vi "Find Salt.vi"(8 "error in (no error)":errorcluster, 11 "Content in":T1) -> (0 "error out":errorcluster, 1 "Salt":string, 2 "BDPW":T3, 3 "Content out":T1)   [LabVIEW 2021, in "VI-Hacker.lvlib"]
uses:
  VI-Hacker.lvlib
  TypeDefs/Content.ctl
  TypeDefs/Block.ctl
  TypeDefs/Block BDPW.ctl
  <vilib>/Utility/error.llb/Error Cluster From Error Code.vi
  <vilib>/ErrorRing/Error Ring.xnode
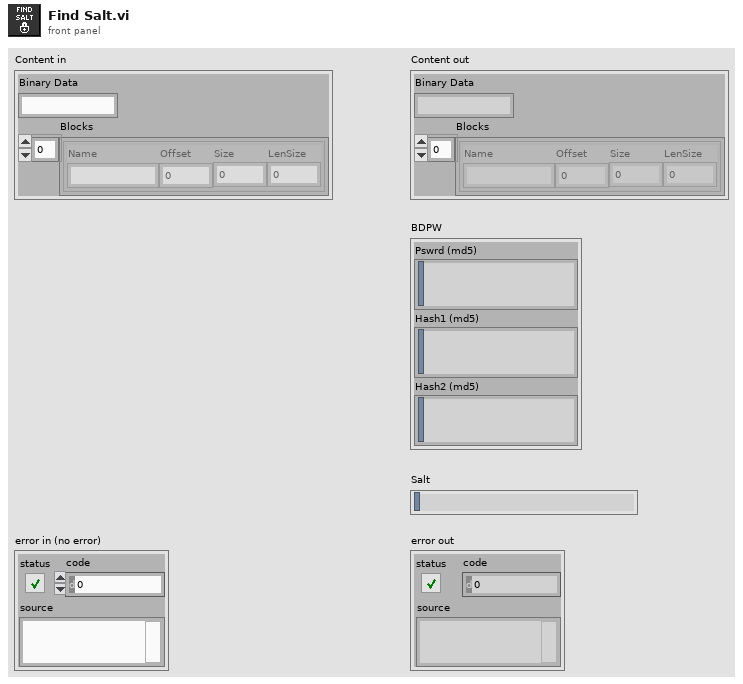
[diagram p1: front panel]
types:
  T1 = typedef "VI-Hacker.lvlib/Content.ctl" = cluster{"Binary Data":string, "Blocks":T2[]}
  T2 = typedef "VI-Hacker.lvlib/Block.ctl" = cluster{"Name":string, "Offset":i32, "Size":i32, "LenSize":i32}
  T3 = typedef "VI-Hacker.lvlib/Block BDPW.ctl" = cluster{"Pswrd (md5)":string, "Hash1 (md5)":string, "Hash2 (md5)":string}
  T4 = typedef "VI-Hacker.lvlib/Block vers.ctl" = cluster{"Version":cluster{"Major":u8, "Minor":u8, "Fix":u8, "Build":u8}, "Stage":enum8{"Development", "Alpha", "Beta", "Release"}, "Flags":u16, "VersionString":string, "VersionInfo":string}
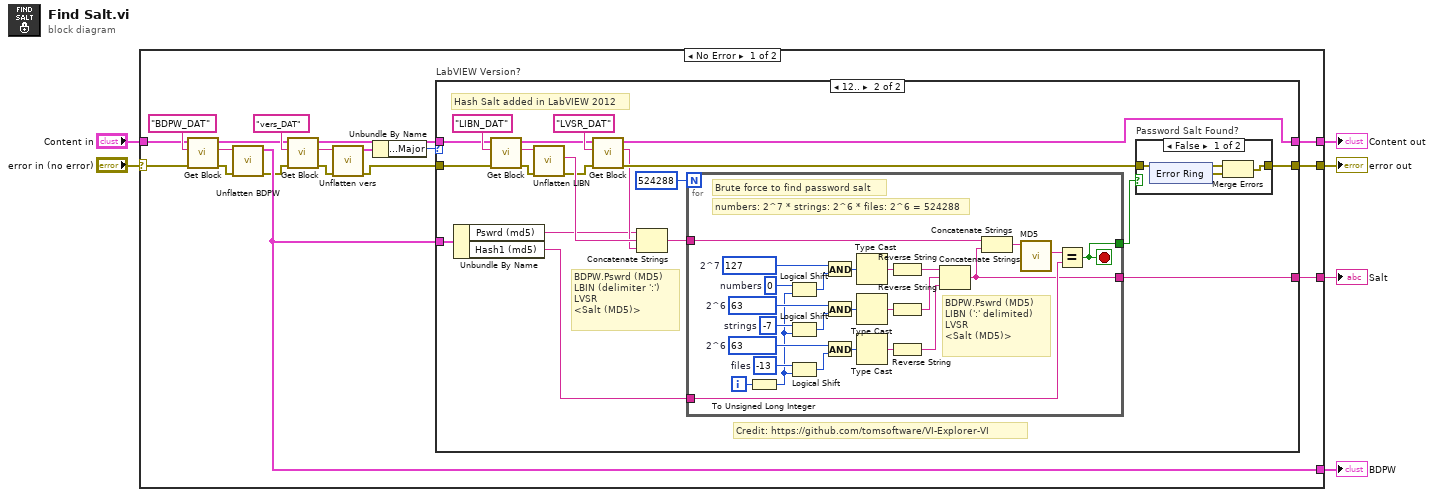
[diagram p0: block diagram]
diagram:
  n1 = case shown="No Error" "error in (no error)" {
    selector: "error in (no error)" -> [w13 w83]
    tunnel: [w24 w83] -> w6
    tunnel: [w23 _] -> w5
    tunnel: [w15 w82] -> w4
    tunnel: [w14 _] -> w3
    tunnel: "Content in" -> [w12 w82]
    frame No Error {
      n2 = call "Get Block.vi"("error in (no error)"=w13, "Block Name"="BDPW_DAT", "Content in"=w12) -> ("error out"=w19:errorcluster, "Data out"=w20:string, "Content out"=w11:T1)  [unwired: 4 in, 2 out]
      n3 = call "Unflatten BDPW.vi"("error in (no error)"=w19, "Data in"=w20) -> ("error out"=w10:errorcluster, "BDPW"=w14:T3)  [unwired: 8 in]
      n4 = call "Get Block.vi"("error in (no error)"=w10, "Block Name"="vers_DAT", "Content in"=w11) -> ("error out"=w18:errorcluster, "Data out"=w17:string, "Content out"=w8:T1)  [unwired: 4 in, 2 out]
      n5 = call "Unflatten vers.vi"("error in (no error)"=w18, "Data in"=w17) -> ("error out"=w9:errorcluster, "vers"=w16:T4)  [unwired: 8 in]
      n6 = Unbundle By Name(w16) -> ("Version.Major"=w7:u8)
      n7 = case "LabVIEW Version?" shown="12.." w7 {
        tunnel: [w26 w46] -> w24
        tunnel: [_ w45] -> w23
        tunnel: [w25 w33] -> w15
        tunnel: w14 -> [_ w32]
        tunnel: w9 -> [w26 w28]
        tunnel: w8 -> [w25 w27]
        frame ..11 {
          # "No salt in LabVIEW 2011 or before"
        }
        frame 12.. {
          # "Credit: https://github.com/tomsoftware/VI-Explorer-VI"
          # "BDPW.Pswrd (MD5)\nLBIN (delimiter ':')\nLVSR\n<Salt (MD5)>"
          # "Hash Salt added in LabVIEW 2012"
          n8 = Unbundle By Name(w32) -> ("Pswrd (md5)"=w35:string, "Hash1 (md5)"=w34:string)
          n9 = call "Get Block.vi"("error in (no error)"=w28, "Block Name"="LIBN_DAT", "Content in"=w27) -> ("error out"=w42:errorcluster, "Data out"=w43:string, "Content out"=w38:T1)  [unwired: 4 in, 2 out]
          n10 = call "Unflatten LIBN.vi"("error in (no error)"=w42, "Data in"=w43) -> ("error out"=w39:errorcluster, "Libraries (MD5 Salt)"=w41:string)  [unwired: 7 in, 1 out]
          n11 = call "Get Block.vi"("error in (no error)"=w39, "Block Name"="LVSR_DAT", "Content in"=w38) -> ("error out"=w37:errorcluster, "Data out"=w36:string, "Content out"=w33:T1)  [unwired: 4 in, 2 out]
          n12 = Concatenate Strings(w35, w41, w36) -> (w30:string)
          n13 = for {
            N: 524288 -> [_]
            tunnel: w30 -> [w81]
            tunnel: w34 -> [w80]
            tunnel: [w71] -> w29
            tunnel: [w58] -> w45
            i -> [w76]
            stop <- w71 stop-if-true
            w69 = u32 63  # 2^6
            w70 = u32 63  # 2^6
            w73 = i8 -13  # files
            w74 = i8 -7  # strings
            w75 = i8 0  # numbers
            w72 = u32 127  # 2^7
            # "numbers: 2^7 * strings: 2^6 * files: 2^6 = 524288"
            # "BDPW.Pswrd (MD5)\nLIBN (':' delimited)\nLVSR\n<Salt (MD5)>"
            # "Brute force to find password salt"
            n14 = To Unsigned Long Integer(number=w76) -> (unsigned 32bit integer=w68:u32)
            n15 = Logical Shift(y=w75, x=w68) -> (x << y=w79:u32)
            n16 = Logical Shift(y=w74, x=w68) -> (x << y=w77:u32)
            n17 = Logical Shift(y=w73, x=w68) -> (x << y=w78:u32)
            n18 = And(x=w72, y=w79) -> (x .and. y?=w64:u32)
            n19 = And(x=w69, y=w77) -> (x .and. y?=w63:u32)
            n20 = And(x=w70, y=w78) -> (x .and. y?=w62:u32)
            n21 = Type Cast(x=w64) -> (*(type *) &x=w67:string)  [unwired: 1 in]
            n22 = Type Cast(x=w63) -> (*(type *) &x=w66:string)  [unwired: 1 in]
            n23 = Type Cast(x=w62) -> (*(type *) &x=w65:string)  [unwired: 1 in]
            n24 = Reverse String(1:w67) -> (0:w61:string)
            n25 = Reverse String(1:w66) -> (0:w60:string)
            n26 = Reverse String(1:w65) -> (0:w59:string)
            n27 = Concatenate Strings(w61, w60, w59) -> (w58:string)
            n28 = Concatenate Strings(w81, w58) -> (w57:string)
            n29 = call "MD5.vi"("Message String"=w57) -> ("MD5 (16-bytes)"=w56:string)  [unwired: 9 in, 1 out]
            n30 = Equal?(x=w56, y=w80) -> (x = y?=w71:bool)
          }
          n31 = case "Password Salt Found?" shown="False" w29 {
            tunnel: w37 -> [w49 w55]
            tunnel: [w48 w55] -> w46
            frame False {
              n32 = xnode "Error Ring"() -> ("error out"=w47:errorcluster)
              n33 = Merge Errors(w49, w47) -> (w48:errorcluster)
            }
            frame True {
            }
          }
        }
      }
    }
    frame Error {
    }
  }
  "error out" <- w6
  "Salt" <- w5
  "BDPW" <- w3
  "Content out" <- w4
